vi "Set Channel.vi"(0 "QCS.lvclass in":refnum<class "QCS.lvclass">, 5 "Channel":u8, 7 "I&R In":T1 {"Current" min=0.0}, 11 "error in (no error)":errorcluster) -> (4 "QCS.lvclass out":refnum<class "QCS.lvclass">, 15 "error out":errorcluster)   [LabVIEW 2016, in "QCS.lvclass"]
uses:
  Lib.llb/QCS.lvclass
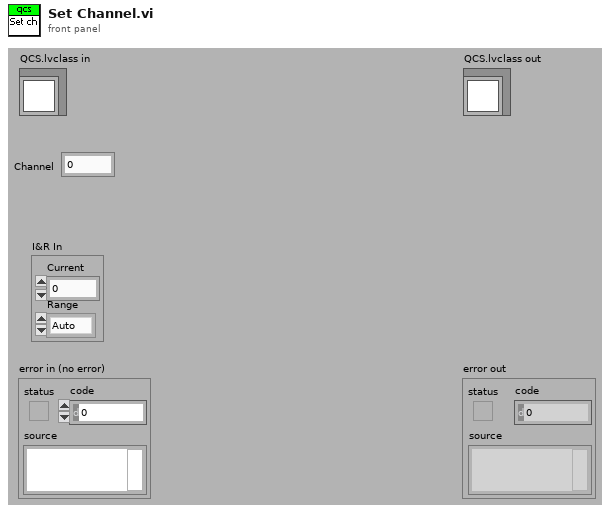
[diagram p1: front panel]
types:
  T1 = cluster{"Current":dbl, "Range":enum8{"Auto", "x1 uA", "x10 uA", "x100 uA", "x1 mA"}}
  T2 = enum8{"Auto", "x1 uA", "x10 uA", "x100 uA", "x1 mA"}
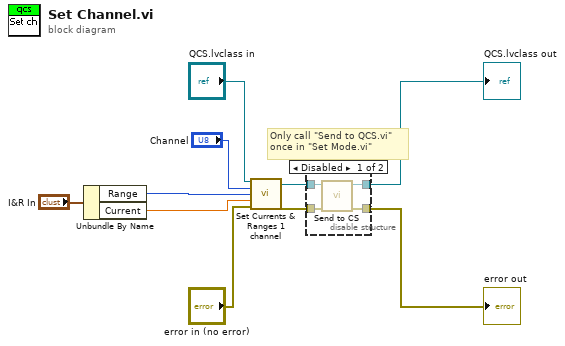
[diagram p0: block diagram]
diagram:
  # "Only call \"Send to QCS.vi\"\nonce in \"Set Mode.vi\""
  n1 = Unbundle By Name("I&R In") -> ("Range"=w6:T2, "Current"=w5:dbl)
  n2 = call-dynamic "Set Currents & Ranges 1 channel.vi"("QCS in"="QCS.lvclass in", "Channel"="Channel", "Range"=w6, "Current"=w5, "error in (no error)"="error in (no error)") -> ("QCS out"=w4:refnum<class "QCS.lvclass">, "error out"=w3:errorcluster)  [unwired: 9 in]
  n3 = disable-structure shown="Disabled" {
    disable-tunnel: w4 -> [w14 w16]
    disable-tunnel: w3 -> [w13 w15]
    disable-tunnel: [w12 w15] -> w2
    disable-tunnel: [w11 w16] -> w1
    frame Disabled {
      n4 = call-dynamic "Send to CS.vi"("error in (no error)"=w13, "QCS in"=w14) -> ("error out"=w12:errorcluster, "QCS out"=w11:refnum<class "QCS.lvclass">)  [unwired: 8 in]
    }
    frame Enabled {
    }
  }
  "error out" <- w2
  "QCS.lvclass out" <- w1
